vi "GetAttributes.vi"(0 "ClassReaderGOOP300 in":refnum<class "ClassReaderGOOP400.lvclass">, 1 "OnlyGetReference":bool, 5 "error in (no error)":errorcluster) -> (14 "ClassReaderGOOP300 out":refnum<class "ClassReaderGOOP400.lvclass">, 15 "ObjectAttributes":T1[](array[typedef])=[{"name"="MyU8", "type"=enum."UINT8", "dimension"=0, "typeName"="", "typePath"=path "", "visibility"=enum."Protected"}, {"name"="MyStrArray", "type"=enum."STRING", "dimension"=1, "typeName"="", "typePath"=path "", "visibility"=enum."Protected"}], 16 "ClassAttributes":T1[](array[typedef])=[{"name"="MyU8", "type"=enum."UINT8", "dimension"=0, "typeName"="", "typePath"=path "", "visibility"=enum."Protected"}, {"name"="MyStrArray", "type"=enum."STRING", "dimension"=1, "typeName"="", "typePath"=path "", "visibility"=enum."Protected"}], 17 "ObjectAttributeReference":refnum<vi>, 18 "ClassAttributeReference":refnum<vi>, 19 "error out":errorcluster)   [LabVIEW 2014, in "ClassReaderGOOP400.lvclass"]
uses:
  <resource>/Framework/Providers/Open_GDS/ClassProviders/Provider_EndevoGOOP400/ClassReaderGOOP400_class/ClassReaderGOOP400.lvclass
  <resource>/Framework/Providers/Open_GDS/UML/ReversedEngineering/ReversedEngineering AttributeInfoType.ctl
  <resource>/Framework/Providers/Open_GDS/ClassProviders/Common/CommonVIs/CommonVIs_AttributeDataType.ctl
  <resource>/Framework/Providers/Open_GDS/UML/UMLEditor/UMLEditor_VisibilityType.ctl
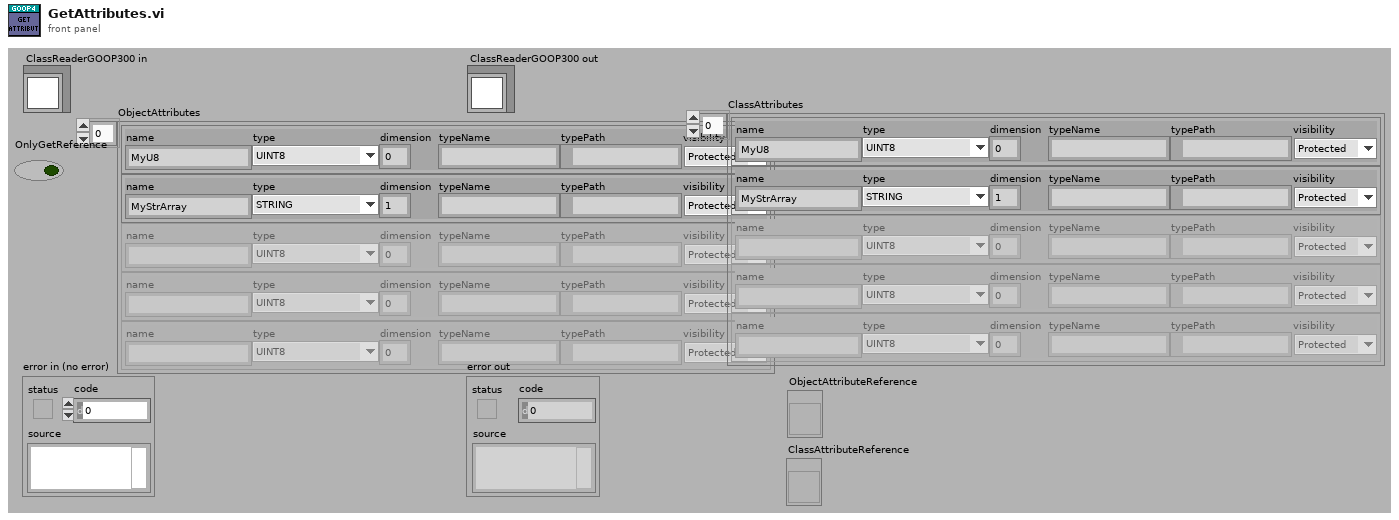
[diagram p1: front panel]
types:
  T1 = typedef "ReversedEngineering AttributeInfoType.ctl" = cluster{"name":string, "type":T2, "dimension":i32, "typeName":string, "typePath":path, "visibility":T3}
  T2 = typedef "CommonVIs_AttributeDataType.ctl" = enum16{"UINT8", "INT8", "UINT16", "INT16", "UINT32", "INT32", "UINT64", "INT64", "SGL", "DBL", "EXT", "CSG", "CDB", "CXT", "TimeStamp", "STRING", "PATH", "BOOL", "ENUM", "RefNum", "VIRefNum", "LabVIEW Class", "Cluster", "Variant", "TypeDef", "Waveform", "LabVIEW Object", "Other", "void"}
  T3 = typedef "UMLEditor_VisibilityType.ctl" = enum16{"Public", "Private", "Protected"}
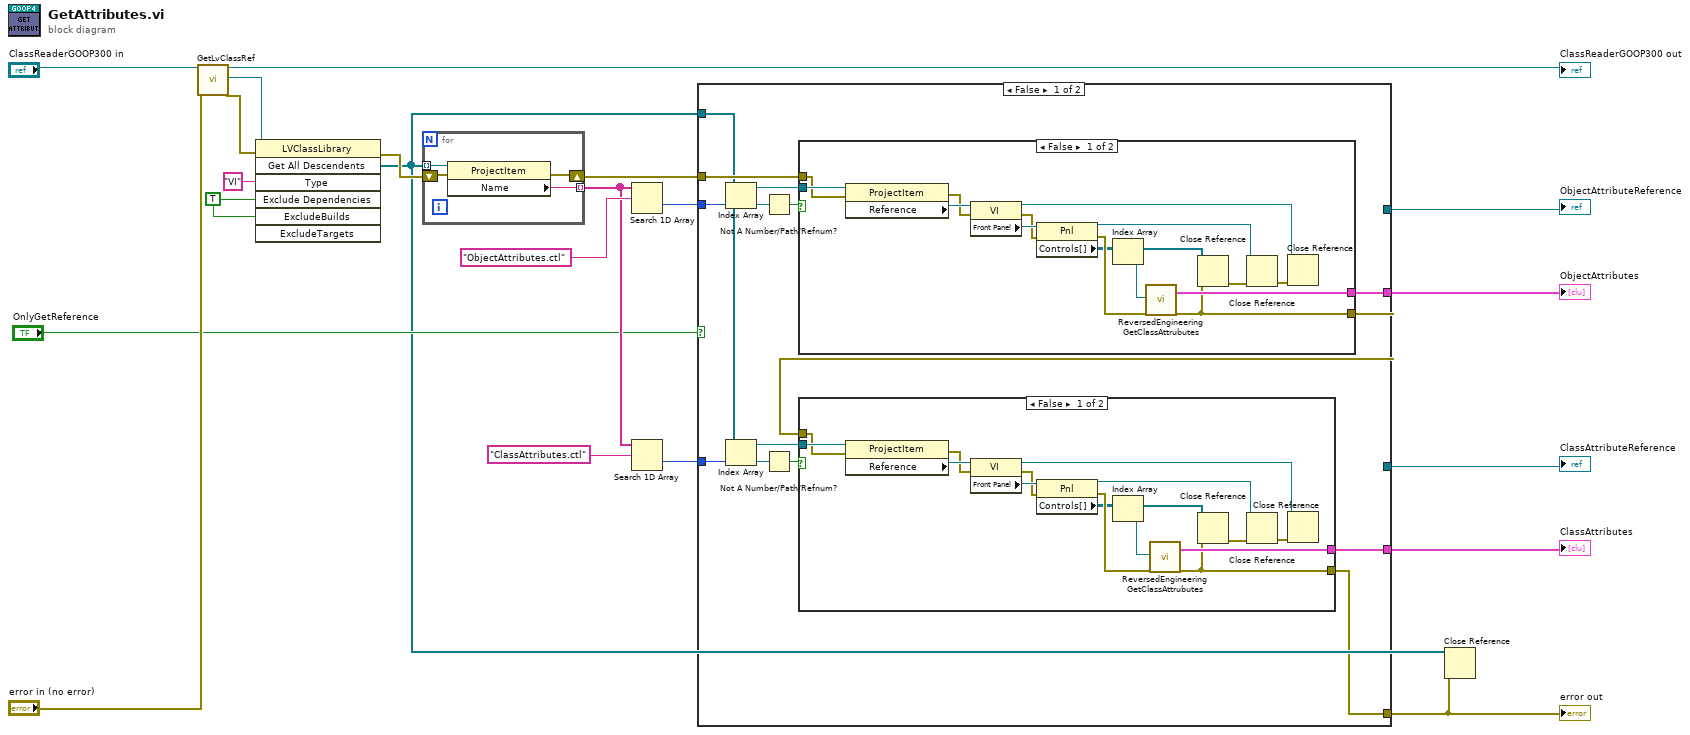
[diagram p0: block diagram]
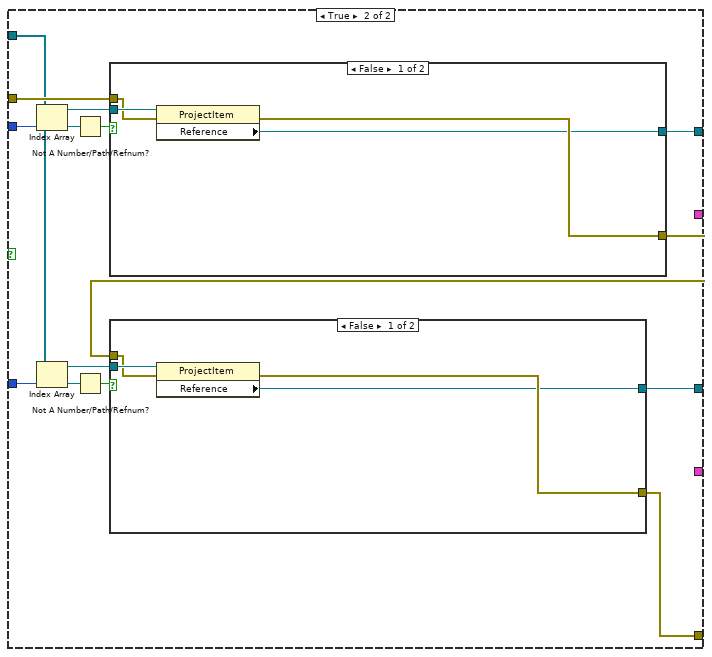
[diagram p4: hidden frame]
diagram:
  w3 = TRUE ("ExcludeDependencies")
  n1 = call-dynamic "GetLvClassRef.vi"("ClassReaderNative in"="ClassReaderGOOP300 in", "error in (no error)"="error in (no error)") -> ("ClassReaderNative out"=→"ClassReaderGOOP300 out":refnum<class "ClassReaderGOOP400.lvclass">, "LvClassRef"=w17:refnum<vi>, "error out"=w14:errorcluster)  [unwired: 15 in]
  n2 = invoke class="LVClassLibrary" method="Get All Descendents"(reference=w17, error in=w14, "Type"="VI", "Exclude Dependencies"=w3, "ExcludeBuilds"=w3) -> (error out=w15:errorcluster, "All Descendents"=w2:refnum<vi>[])  [unwired: 2 in, 5 out]
  n3 = for {
    tunnel: w2 -> [w25] mode=indexing
    tunnel: [w24] -> w11 mode=indexing
    shift-right: [w22] -> w12
    shift-left: w15 -> [w23]
    n4 = property class="ProjectItem"(reference=w25, error in=w23) -> (error out=w22:errorcluster, "Name"=w24:string)  [unwired: 1 out]
  }
  n5 = Search 1D Array(1D array=w11, element="ObjectAttributes.ctl" ("string")) -> (index of element=w8:i32)  [unwired: 1 in]
  n6 = Search 1D Array(1D array=w11, element="ClassAttributes.ctl" ("string")) -> (index of element=w7:i32)  [unwired: 1 in]
  n7 = case shown="False" "OnlyGetReference" {
    tunnel: [w37 _] -> w19
    tunnel: w12 -> [w35 w80]
    tunnel: [w30 _] -> w9
    tunnel: [w29 w75] -> w1
    tunnel: w2 -> [w28 w74]
    tunnel: w8 -> [w27 w73]
    tunnel: w7 -> [w26 w72]
    tunnel: [_ w71] -> w5
    tunnel: [_ w70] -> w4
    frame False {
      n8 = Index Array(array=w28, index=w27) -> (element=w36:refnum<vi>)
      n9 = Index Array(array=w28, index=w26) -> (element=w32:refnum<vi>)
      n10 = Not A Number/Path/Refnum?(number/path/refnum=w36) -> (NaN/Path/Refnum?=w34:bool)
      n11 = Not A Number/Path/Refnum?(number/path/refnum=w32) -> (NaN/Path/Refnum?=w33:bool)
      n12 = case shown="False" w34 {
        tunnel: [w68 _] -> w37
        tunnel: w36 -> [w67 _]
        tunnel: w35 -> [w62 w69]
        tunnel: [w58 w69] -> w31
        frame False {
          n13 = property class="ProjectItem"(reference=w67, error in=w62) -> (error out=w63:errorcluster, "Reference"=w64:refnum<vi>)  [unwired: 1 out]
          n14 = property class="VI"(reference=w64, error in=w63) -> (reference out=w55:refnum<vi>, error out=w65:errorcluster, "Front Panel"=w66:refnum<vi>)
          n15 = property class="Pnl"(reference=w66, error in=w65) -> (reference out=w57:refnum<vi>, error out=w61:errorcluster, "Controls[]"=w54:refnum<vi>[])
          n16 = Index Array(array=w54) -> (element=w60:refnum<vi>)  [unwired: 1 in]
          n17 = call <resource>:"ReversedEngineering GetClassAttrubutes.vi"("CtlRefnum"=w60, "error in (no error)"=w61) -> ("attributeInfo"=w68:T1[], "error out"=w58:errorcluster)  [unwired: 15 in, 1 out]
          n18 = Close Reference(reference=w54, error in (no error)=w58) -> (error out=w59:errorcluster)
          n19 = Close Reference(reference=w57, error in (no error)=w59) -> (error out=w56:errorcluster)
          n20 = Close Reference(reference=w55, error in (no error)=w56) -> ()  [unwired: 1 out]
        }
        frame True {
        }
      }
      n21 = case shown="False" w33 {
        tunnel: [w52 _] -> w30
        tunnel: w32 -> [w51 _]
        tunnel: w31 -> [w46 w53]
        tunnel: [w41 w53] -> w29
        frame False {
          n22 = property class="ProjectItem"(reference=w51, error in=w46) -> (error out=w47:errorcluster, "Reference"=w48:refnum<vi>)  [unwired: 1 out]
          n23 = property class="VI"(reference=w48, error in=w47) -> (reference out=w39:refnum<vi>, error out=w49:errorcluster, "Front Panel"=w50:refnum<vi>)
          n24 = property class="Pnl"(reference=w50, error in=w49) -> (reference out=w40:refnum<vi>, error out=w45:errorcluster, "Controls[]"=w38:refnum<vi>[])
          n25 = Index Array(array=w38) -> (element=w42:refnum<vi>)  [unwired: 1 in]
          n26 = call <resource>:"ReversedEngineering GetClassAttrubutes.vi"("CtlRefnum"=w42, "error in (no error)"=w45) -> ("attributeInfo"=w52:T1[], "error out"=w41:errorcluster)  [unwired: 15 in, 1 out]
          n27 = Close Reference(reference=w38, error in (no error)=w41) -> (error out=w43:errorcluster)
          n28 = Close Reference(reference=w40, error in (no error)=w43) -> (error out=w44:errorcluster)
          n29 = Close Reference(reference=w39, error in (no error)=w44) -> ()  [unwired: 1 out]
        }
        frame True {
        }
      }
    }
    frame True {
      n30 = Index Array(array=w74, index=w73) -> (element=w81:refnum<vi>)
      n31 = Index Array(array=w74, index=w72) -> (element=w77:refnum<vi>)
      n32 = Not A Number/Path/Refnum?(number/path/refnum=w81) -> (NaN/Path/Refnum?=w79:bool)
      n33 = Not A Number/Path/Refnum?(number/path/refnum=w77) -> (NaN/Path/Refnum?=w78:bool)
      n34 = case shown="False" w79 {
        tunnel: w81 -> [w90 _]
        tunnel: w80 -> [w89 w91]
        tunnel: [w88 w91] -> w76
        tunnel: [w87 _] -> w71
        frame False {
          n35 = property class="ProjectItem"(reference=w90, error in=w89) -> (error out=w88:errorcluster, "Reference"=w87:refnum<vi>)  [unwired: 1 out]
        }
        frame True {
        }
      }
      n36 = case shown="False" w78 {
        tunnel: w77 -> [w85 _]
        tunnel: w76 -> [w84 w86]
        tunnel: [w83 w86] -> w75
        tunnel: [w82 _] -> w70
        frame False {
          n37 = property class="ProjectItem"(reference=w85, error in=w84) -> (error out=w83:errorcluster, "Reference"=w82:refnum<vi>)  [unwired: 1 out]
        }
        frame True {
        }
      }
    }
  }
  "ObjectAttributes" <- w19
  "ClassAttributes" <- w9
  "error out" <- w1
  "ClassAttributeReference" <- w4
  "ObjectAttributeReference" <- w5
  n38 = Close Reference(reference=w2, error in (no error)=w1) -> ()  [unwired: 1 out]
